vi "dfd_Convert Waveform Graph to XY Graph (Single Graph).vi"(10 "waveform":cluster{"f0":dbl, "df":dbl, "values":dbl[]}) -> (2 "XY graph":cluster{dbl[], "values":dbl[]})   [LabVIEW 2017, in "NI_DigFilter_FilterBank.lvlib"]
uses:
  <vilib>/addons/Digital Filter Design/NI_DigFilter_FilterBank.lvlib
  <vilib>/Analysis/1siggen.llb/Ramp Pattern by Samples.vi
  <vilib>/Analysis/NI_AALBase.lvlib
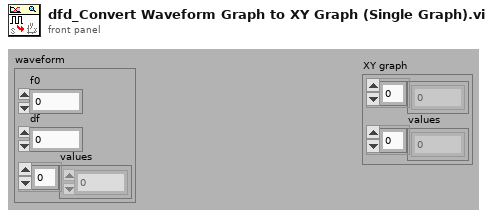
[diagram p1: front panel]
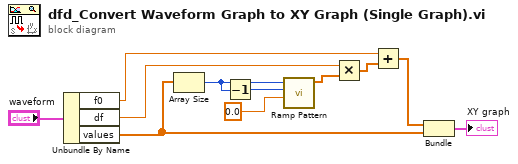
[diagram p0: block diagram]
diagram:
  n1 = Unbundle By Name("waveform") -> ("f0"=w2:dbl, "df"=w4:dbl, "values"=w11:dbl[])
  n2 = Array Size(array=w11) -> (size(s)=w7:i32)
  n3 = Decrement(x=w7) -> (x-1=w8:i32)
  n4 = call-poly <vilib>:"Ramp Pattern.vi"("start"=0.0, "end"=w8, "samples"=w7) -> ("Ramp Pattern"=w5:dbl[])  [unwired: 7 in, 1 out]
  n5 = Multiply(x=w4, y=w5) -> (x*y=w3:dbl[])
  n6 = Add(x=w2, y=w3) -> (x+y=w1:dbl[])
  n7 = Bundle(w1, "values"=w11) -> (→"XY graph":cluster{dbl[], "values":dbl[]})  [unwired: 1 in]
